vi "Begin-Finish.vi"(11 "Enum":enum16{"Start", "Run", "End"}(ring)) -> ()   [LabVIEW 2014]
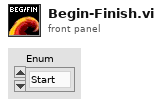
[diagram p1: front panel]
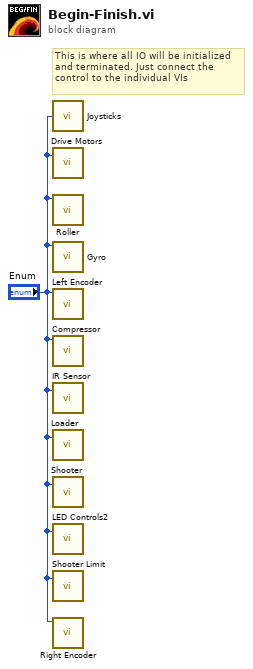
[diagram p0: block diagram]
diagram:
  # "This is where all IO will be initialized\nand terminated. Just connect the \ncontrol to the individual VIs"
  n1 = call "Joysticks.vi"("Enum"="Enum") -> ()  [unwired: 2 out]
  n2 = call "Drive Motors.vi"("Enum"="Enum") -> ()  [unwired: 1 in]
  n3 = call "Roller.vi"("Enum"="Enum") -> ()  [unwired: 3 in]
  n4 = call "Gyro.vi"("Enum"="Enum") -> ()  [unwired: 10 in, 1 out]
  n5 = call "Left Encoder.vi"("Enum"="Enum") -> ()  [unwired: 9 in, 2 out]
  n6 = call "Compressor.vi"("Enum"="Enum") -> ()  [unwired: 11 in]
  n7 = call "IR Sensor.vi"("Enum"="Enum") -> ()  [unwired: 1 in, 1 out]
  n8 = call "Loader.vi"("Enum"="Enum") -> ()  [unwired: 1 in, 1 out]
  n9 = call "Shooter.vi"("Enum"="Enum") -> ()  [unwired: 2 in]
  n10 = call "LED Controls2.vi"("Enum"="Enum") -> ()  [unwired: 2 in]
  n11 = call "Shooter Limit.vi"("Enum"="Enum") -> ()  [unwired: 1 in, 1 out]
  n12 = call "Right Encoder.vi"("Enum"="Enum") -> ()  [unwired: 9 in, 2 out]
